vi "Prepare Acquisition.vi"(8 "error in (no error)":errorcluster, 10 "Camera Settings":T1={"Exposure Time (ms)"=100.0, "Binning"=enum."2x2", "Scan Mode"=0, "Frames to Acquire"=1000.0, "Pixel Correction"=FALSE, "Frames to Skip"=0, "File Path"=path "", "Duty cycle"=0.0, "ALEX"=FALSE, "Shutter Enable"=[], "fluidics trigger frame"=0, "Bit Depth"=0, "Image Width (px)"=0, "Image Height (px)"=0, "Horizontal Offset (px)"=0, "Vertical Offset (px)"=0} {"fluidics trigger frame" max=60000 step=1; "Exposure Time (ms)" min=1.0 max=10000.0 step=1.0}, 11 "Andor Camera in":refnum<class "Andor Camera.lvclass">) -> (0 "error out":errorcluster, 3 "Andor Camera out":refnum<class "Andor Camera.lvclass">)   [LabVIEW 2018, in "Andor Camera.lvlib" / "Andor Camera.lvclass"]
uses:
  Andor Camera.lvclass
  Resources/Type Defs/Camera Settings.ctl
  <userlib>/atmcd64d.llb/ReadMode_mode typedef.ctl
  <userlib>/atmcd64d.llb/TriggerMode_mode typedef.ctl
panel:
  out "FT":sgl
  out "Valid exposure":sgl format="%.2f"
  out "Frame time error (ms)":dbl
  out "Valid Cycle time":sgl format="%.4f"
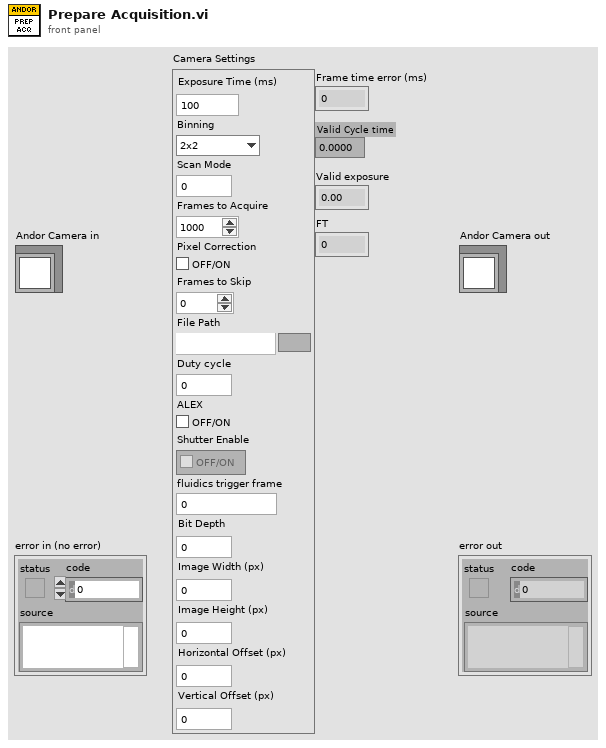
[diagram p1: front panel]
types:
  T1 = typedef "Camera Settings.ctl" = cluster{"Exposure Time (ms)":dbl, "Binning":enum16{"1x1", "2x2", "4x4"}, "Scan Mode":i32, "Frames to Acquire":dbl, "Pixel Correction":bool, "Frames to Skip":u32, "File Path":path, "Duty cycle":dbl, "ALEX":bool, "Shutter Enable":bool[], "fluidics trigger frame":u16, "Bit Depth":u16, "Image Width (px)":u16, "Image Height (px)":u16, "Horizontal Offset (px)":u16, "Vertical Offset (px)":u16}
  T2 = typedef "ReadMode_mode typedef.ctl" = enum16{"Full Vertical Binning", "Multi-Track", "Random-Track", "Single-Track", "Image"}
  T3 = typedef "TriggerMode_mode typedef.ctl" = enum16{"Internal", "External", "N/A (2)", "N/A (3)", "N/A (4)", "N/A (5)", "External Start", "External Exposure (Bulb)", "N/A (8)", "External FVB EM", "Software", "N/A (11)", "External Charge Shifting"}
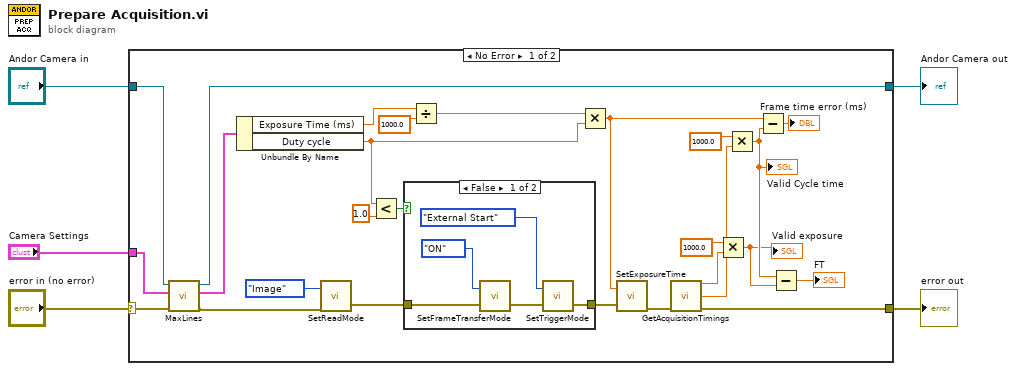
[diagram p0: block diagram]
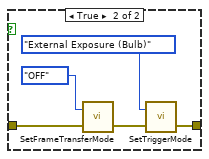
[diagram p2: hidden frame]
diagram:
  n1 = case shown="No Error" "error in (no error)" {
    selector: "error in (no error)" -> [w28 w43]
    tunnel: [w31 w43] -> w4
    tunnel: [w22 w42] -> w2
    tunnel: "Andor Camera in" -> [w23 w42]
    tunnel: "Camera Settings" -> [w26 _]
    frame No Error {
      n2 = call-dynamic "MaxLines.vi"("error in (no error)"=w28, "Camera Settings"=w26, "Andor Camera in"=w23) -> ("error out"=w27:errorcluster, "Camera Settings 2"=w25:T1, "Andor Camera out"=w22:refnum<class "Andor Camera.lvclass">)  [unwired: 6 in]
      n3 = Unbundle By Name(w25) -> ("Exposure Time (ms)"=w7:dbl, "Duty cycle"=w10:dbl)
      n4 = call <userlib>:"SetReadMode.vi"("error in (no error)"=w27, "mode"=ReadMode_mode_typedef."Image") -> ("error out"=w12:errorcluster)  [unwired: 1 out]
      n5 = Less?(x=w10, y=1.0) -> (x < y?=w21:bool)
      n6 = case shown="False" w21 {
        tunnel: w12 -> [w32 w41]
        tunnel: [w33 w37] -> w11
        frame False {
          n7 = call <userlib>:"SetFrameTransferMode.vi"("error in (no error)"=w32, "mode"=enum16{"OFF", "ON"}."ON") -> ("error out"=w35:errorcluster)  [unwired: 1 out]
          n8 = call <userlib>:"SetTriggerMode.vi"("error in (no error)"=w35, "mode"=TriggerMode_mode_typedef."External Start") -> ("error out"=w33:errorcluster)  [unwired: 1 out]
        }
        frame True {
          n9 = call <userlib>:"SetFrameTransferMode.vi"("error in (no error)"=w41, "mode"=enum16{"OFF", "ON"}."OFF") -> ("error out"=w39:errorcluster)  [unwired: 1 out]
          n10 = call <userlib>:"SetTriggerMode.vi"("error in (no error)"=w39, "mode"=TriggerMode_mode_typedef."External Exposure (Bulb)") -> ("error out"=w37:errorcluster)  [unwired: 1 out]
        }
      }
      n11 = Divide(x=w7, y=1000.0) -> (x/y=w6:dbl)
      n12 = Multiply(x=w6, y=w10) -> (x*y=w8:dbl)
      n13 = call <userlib>:"SetExposureTime.vi"("error in (no error)"=w11, "time"=w8) -> ("error out"=w30:errorcluster)  [unwired: 1 out]
      n14 = call <userlib>:"GetAcquisitionTimings.vi"("error in (no error)"=w30) -> ("exposure"=w16:sgl, "kinetic"=w18:sgl, "error out"=w31:errorcluster)  [unwired: 10 in, 2 out]
      n15 = Multiply(x=sgl 1000.0 ("y"), y=w16) -> (x*y=w14:sgl)
      "Valid exposure" <- w14
      n16 = Multiply(x=sgl 1000.0 ("y"), y=w18) -> (x*y=w15:sgl)
      "Valid Cycle time" <- w15
      n17 = Subtract(x=w8, y=w15) -> (x-y=→"Frame time error (ms)":dbl)
      n18 = Subtract(x=w15, y=w14) -> (x-y=→"FT":sgl)
    }
    frame Error {
    }
  }
  "error out" <- w4
  "Andor Camera out" <- w2
